vi "NumericCaseString.vi"(5 "selector string":string, 8 "data type":variant) -> (1 "Default":bool, 4 "case":string)   [LabVIEW 2014, in "CaseStructure.lvclass"]
uses:
  CaseStructure.lvclass
  Python/Parsing/ListTypesTD.ctl
  Python/Parsing/Python Functions.lvlib
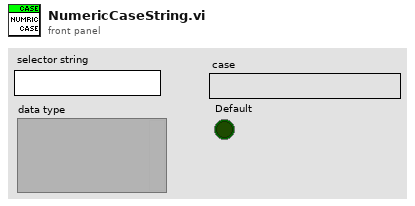
[diagram p1: front panel]
types:
  T1 = typedef "Python Functions.lvlib/ListTypesTD.ctl" = enum16{"list", "tuple", "parameter list", "output list", "return values"}
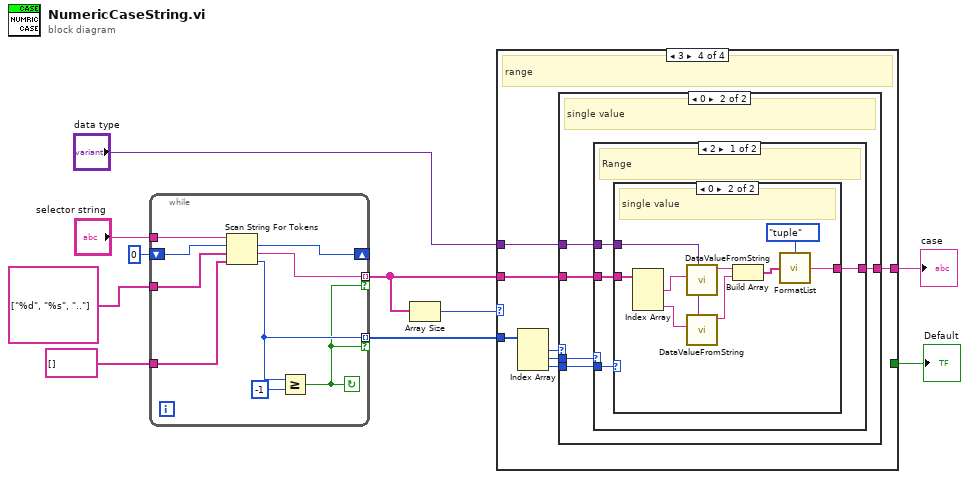
[diagram p0: block diagram]
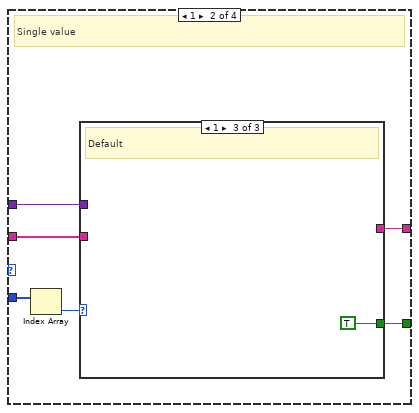
[diagram p3: hidden frame]
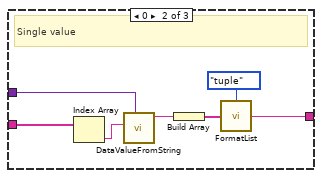
[diagram p5: hidden frame]
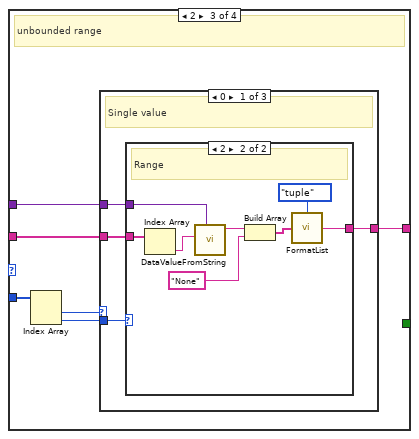
[diagram p6: hidden frame]
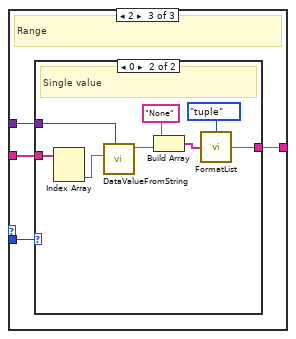
[diagram p9: hidden frame]
diagram:
  n1 = while {
    tunnel: "selector string" -> [w19]
    shift-right: [w17] -> _
    shift-left: 0 ("offset past token") -> [w18]
    tunnel: string[] [] ("delimiters (\\s,\\t,\\r,\\n)") -> [w16]
    tunnel: [w15] -> w5 mode=indexing if=w11
    tunnel: string[] ["%d", "%s", ".."] ("operators (none)") -> [w14]
    tunnel: [w13] -> w4 mode=indexing if=w11
    stop <- w11 continue-if-true
    n2 = Scan String For Tokens(6:w16, 7:w14, 8:w18, 9:w19) -> (0:w13:i32, 1:w15:string, 2:w17:i32)  [unwired: 2 in, 1 out]
    n3 = Greater Or Equal?(x=w13, y=-1) -> (x >= y?=w11:bool)
  }
  n4 = Array Size(array=w5) -> (size(s)=w6:i32)
  n5 = case shown="3" w6 {
    tunnel: w5 -> [_ w25 w39 w70]
    tunnel: [_ w24 w38 w69] -> w3
    tunnel: w4 -> [_ w23 w37 w68]
    tunnel: "data type" -> [_ w21 w34 w65]
    tunnel: [_ w20 _ _] -> w2
    frame Default {
      # "Error"
    }
    frame 1 {
      # "Single value"
      n6 = Index Array(array=w23) -> (element=w22:i32)  [unwired: 1 in]
      n7 = case shown="1" w22 {
        tunnel: w25 -> [_ w31 _]
        tunnel: [_ w27 _] -> w24
        tunnel: w21 -> [_ w26 _]
        tunnel: [_ _ TRUE] -> w20
        frame Default {
          # "Error"
        }
        frame 0 {
          # "Single value"
          n8 = Index Array(array=w31) -> (element=w30:string)  [unwired: 1 in]
          n9 = call "DataValueFromString.vi"("Type"=w26, "value"=w30) -> ("value"=w28:string)  [unwired: 7 in]
          n10 = Build Array(w28) -> (w29:string[])
          n11 = call "FormatList.vi"("values"=w29, "type"=ListTypesTD."tuple") -> ("python object"=w27:string)
        }
        frame 1 {
          # "Default"
        }
      }
    }
    frame 2 {
      # "unbounded range"
      n12 = Index Array(array=w37) -> (element #1=w35:i32, element #2=w36:i32)  [unwired: 2 in]
      n13 = case shown="0" w35 {
        tunnel: w39 -> [w43 _ w55]
        tunnel: [w42 _ w54] -> w38
        tunnel: w36 -> [w41 _ w53]
        tunnel: w34 -> [w40 _ w52]
        frame 0 {
          # "Single value"
          n14 = case shown="2" w41 {
            tunnel: w43 -> [_ w50]
            tunnel: [_ w46] -> w42
            tunnel: w40 -> [_ w44]
            frame Default {
              # "Error"
            }
            frame 2 {
              # "Range"
              n15 = Index Array(array=w50) -> (element=w49:string)  [unwired: 1 in]
              n16 = call "DataValueFromString.vi"("Type"=w44, "value"=w49) -> ("value"=w47:string)  [unwired: 7 in]
              n17 = Build Array(w47, "None" ("element")) -> (w48:string[])
              n18 = call "FormatList.vi"("values"=w48, "type"=ListTypesTD."tuple") -> ("python object"=w46:string)
            }
          }
        }
        frame Default {
          # "Error"
        }
        frame 2 {
          # "Range"
          n19 = case shown="0" w53 {
            tunnel: w55 -> [_ w62]
            tunnel: [_ w59] -> w54
            tunnel: w52 -> [_ w57]
            frame Default {
              # "Error"
            }
            frame 0 {
              # "Single value"
              n20 = Index Array(array=w62) -> (element #2=w56:string)  [unwired: 2 in, 1 out]
              n21 = call "DataValueFromString.vi"("Type"=w57, "value"=w56) -> ("value"=w60:string)  [unwired: 7 in]
              n22 = Build Array("None" ("element"), w60) -> (w61:string[])
              n23 = call "FormatList.vi"("values"=w61, "type"=ListTypesTD."tuple") -> ("python object"=w59:string)
            }
          }
        }
      }
    }
    frame 3 {
      # "range"
      n24 = Index Array(array=w68) -> (element #1=w64:i32, element #2=w66:i32, element #3=w67:i32)  [unwired: 3 in]
      n25 = case shown="0" w64 {
        tunnel: w70 -> [_ w75]
        tunnel: [_ w74] -> w69
        tunnel: w67 -> [_ w73]
        tunnel: w66 -> [_ w72]
        tunnel: w65 -> [_ w71]
        frame Default {
          # "error"
        }
        frame 0 {
          # "single value"
          n26 = case shown="2" w72 {
            tunnel: w75 -> [w79 _]
            tunnel: [w78 _] -> w74
            tunnel: w73 -> [w77 _]
            tunnel: w71 -> [w76 _]
            frame 2 {
              # "Range"
              n27 = case shown="0" w77 {
                tunnel: w79 -> [_ w87]
                tunnel: [_ w83] -> w78
                tunnel: w76 -> [_ w82]
                frame Default {
                  # "Error"
                }
                frame 0 {
                  # "single value"
                  n28 = Index Array(array=w87) -> (element #1=w86:string, element #3=w80:string)  [unwired: 3 in, 1 out]
                  n29 = call "DataValueFromString.vi"("Type"=w82, "value"=w86) -> ("value"=w84:string)  [unwired: 7 in]
                  n30 = call "DataValueFromString.vi"("Type"=w82, "value"=w80) -> ("value"=w81:string)  [unwired: 7 in]
                  n31 = Build Array(w84, w81) -> (w85:string[])
                  n32 = call "FormatList.vi"("values"=w85, "type"=ListTypesTD."tuple") -> ("python object"=w83:string)
                }
              }
            }
            frame Default {
              # "Error"
            }
          }
        }
      }
    }
  }
  "case" <- w3
  "Default" <- w2
